vi "Boradcat All Notifier.vi"(7 "Timeout":i32=-1, 8 "error in (no error)":errorcluster, 10 "Notification In":variant, 11 "Simple Map Notifier Controller in":refnum<class "Simple Map SEQ I64 Notifier Controller.lvclass">) -> (0 "error out":errorcluster, 3 "Simple Map Notifier Controller out":refnum<class "Simple Map SEQ I64 Notifier Controller.lvclass">)   [LabVIEW 2019, in "Simple Map SEQ I64 Notifier Controller.lvclass"]
uses:
  Simple Map SEQ I64 Notifier Controller.lvclass
  Simple Map SEQ I64 Notifier Controller.lvclass/Simple Map SEQ I64 Notifier Controller.ctl
  Ancestor Class/Actor Assistant/Notifier/Notifier.lvclass
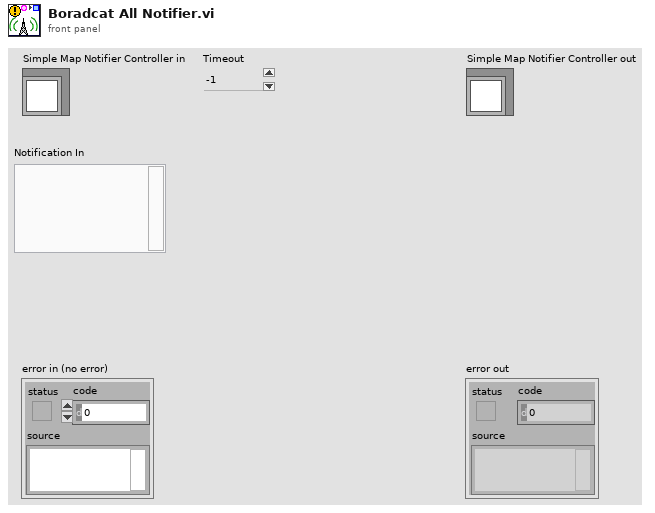
[diagram p1: front panel]
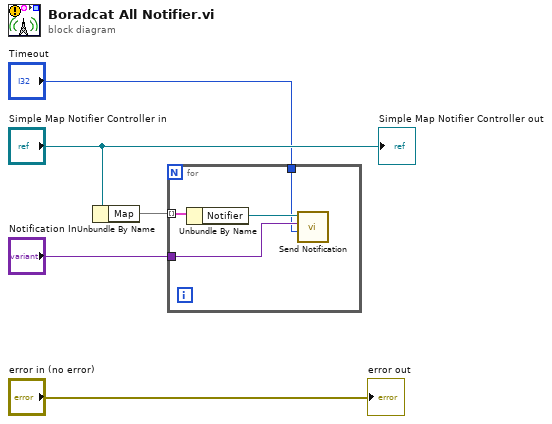
[diagram p0: block diagram]
diagram:
  n1 = Unbundle By Name("Simple Map Notifier Controller in") -> ("Map"=w3:map{i64, refnum<class "Notifier.lvclass">})
  n2 = for {
    tunnel: w3 -> [w9] mode=indexing
    tunnel: "Notification In" -> [w7]
    tunnel: "Timeout" -> [w6]
    n3 = Unbundle By Name(w9) -> ("Notifier"=w8:refnum<class "Notifier.lvclass">)
    n4 = call-dynamic "Send Notification.vi"("Timeout"=w6, "Notification"=w7, "Notifier in"=w8) -> ()  [unwired: 6 in, 3 out]
  }
  "error out" <- "error in (no error)"
  "Simple Map Notifier Controller out" <- "Simple Map Notifier Controller in"
